vi "Save Animated GIF Image (Path).vi"(6 "Loop Count (forever)":i32, 8 "error in (no error)":errorcluster, 9 "Delays":i32[](array[numeric]), 10 "Frames":T1[](array[typedef]), 11 "Path In":path) -> (0 "error out":errorcluster, 3 "Path Out":path)   [LabVIEW 2020, in "G-Image.lvlib"]
doc: "Saves a series of images in animated GIF format to disk.\n\nIf the input images have an alpha channel or mask, they will be used to set the transparent pixels of the resulting animated GIF.\n\n<b>Loop Count</b> sets the number of times the animation will play before looping, where 0 means loop forever."
uses:
  G-Image.lvlib
  <vilib>/picture/picture.llb/imagedata.ctl
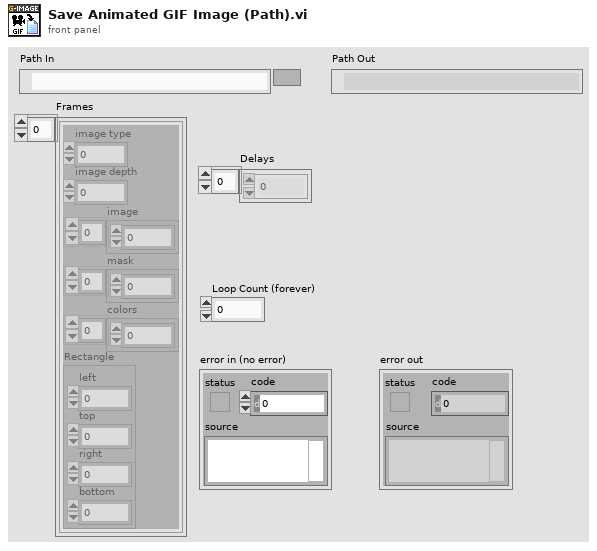
[diagram p1: front panel]
types:
  T1 = typedef "imagedata.ctl" = cluster{"image type":i32, "image depth":i32, "image":u8[], "mask":u8[], "colors":u32[], "Rectangle":cluster{"left":i16, "top":i16, "right":i16, "bottom":i16}}
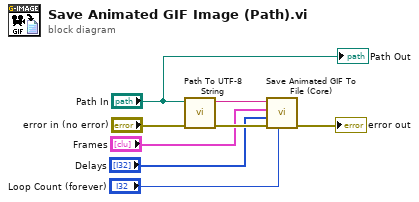
[diagram p0: block diagram]
diagram:
  n1 = call "Path To UTF-8 String.vi"("error in"="error in (no error)", "Path"="Path In") -> ("error out"=w4:errorcluster, "UTF-8 String"=w7:string)  [unwired: 8 in]
  n2 = call "Save Animated GIF To File (Core).vi"("Loop Count (forever)"="Loop Count (forever)", "error in (no error)"=w4, "Delays"="Delays", "Frames"="Frames", "Path In"=w7) -> ("error out"=→"error out":errorcluster)  [unwired: 5 in, 1 out]
  "Path Out" <- "Path In"
